vi "XNETDB.Add.vi"(8 "error in (no error)":errorcluster, 11 "Databases Section Ref":T1 format="%.0x") -> (0 "error out":errorcluster, 3 "Databases Section Ref":u64)   [LabVIEW 2019, in "Diagnostics Addon Shared.lvlib"]
uses:
  Diagnostics Addon Shared.lvlib
  <vilib>/NI VeriStand/Custom Device API/Custom Device Item Ref.ctl
  Constants.vi
  <vilib>/NI/NI VeriStand Advanced SysDef API/_SubVIs/SysDef.Property.Set.String.vi
  <vilib>/NI/NI VeriStand Advanced SysDef API/SysDef API/Advanced System Definition.lvlib
  <vilib>/NI VeriStand/Custom Device API/Custom Device API.lvlib
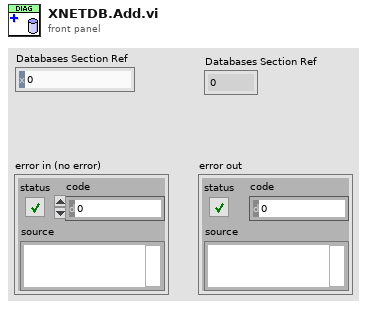
[diagram p1: front panel]
types:
  T1 = typedef "Custom Device API.lvlib/Custom Device Item Ref.ctl" = u64
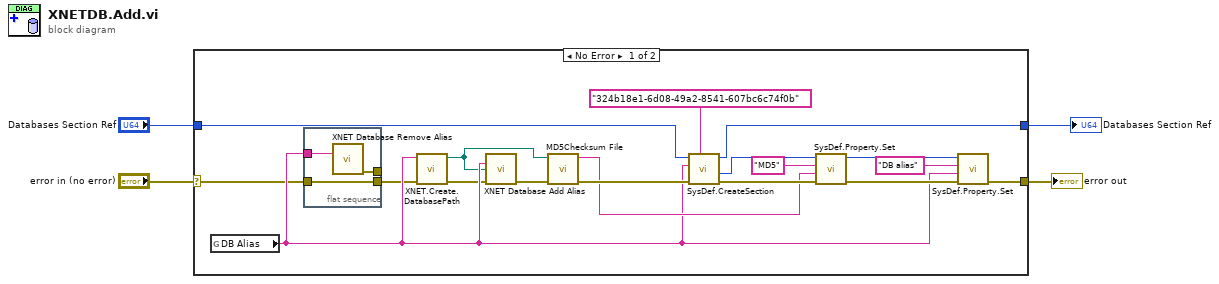
[diagram p0: block diagram]
diagram:
  n1 = case shown="No Error" "error in (no error)" {
    selector: "error in (no error)" -> [w6 w27]
    tunnel: "Databases Section Ref" -> [w22 w26]
    tunnel: [w21 w27] -> w3
    tunnel: [w5 w26] -> w1
    frame No Error {
      n2 = global read "Constants.vi" "DB Alias"() -> (w10:string)
      n3 = flat-sequence {
        tunnel: [w25] -> w8
        tunnel: w6 -> [w25]
        tunnel: [w24] -> _
        tunnel: w10 -> [w23]
        frame #0 {
          n4 = call <vilib>:"XNET Database Remove Alias.vi"("alias"=w23) -> ("error out"=w24:errorcluster)  [unwired: 14 in]
        }
      }
      n5 = call "XNET.Create.DatabasePath.vi"("error in (no error)"=w8, "DB Alias"=w10) -> ("error out"=w9:errorcluster, "DB Path"=w7:path)  [unwired: 8 in]
      n6 = call <vilib>:"XNET Database Add Alias.vi"("alias"=w10, "filepath"=w7, "error in (no error)"=w9) -> ("error out"=w20:errorcluster)  [unwired: 12 in]
      n7 = call <vilib>:"MD5Checksum File.vi"("error in (no error)"=w20, "Path"=w7) -> ("error out"=w12:errorcluster, "MD5 message-digest"=w11:string)  [unwired: 8 in]
      n8 = call <vilib>:"SysDef.CreateSection.vi"("GUID"="324b18e1-6d08-49a2-8541-607bc6c74f0b" ("GUID (Default Section)"), "error in (no error)"=w12, "Name"=w10, "nodeID"=w22) -> ("error out"=w18:errorcluster, "New NodeID"=w19:u64, "nodeID out"=w5:u64)  [unwired: 4 in, 1 out]
      n9 = call-poly <vilib>:"SysDef.Property.Set.vi"("error in (no error)"=w18, "Value"=w11, "Property Name"="MD5", "nodeID"=w19) -> ("error out"=w17:errorcluster, "nodeID out"=w16:u64)  [unwired: 6 in]
      n10 = call-poly <vilib>:"SysDef.Property.Set.vi"("error in (no error)"=w17, "Value"=w10, "Property Name"="DB alias", "nodeID"=w16) -> ("error out"=w21:errorcluster)  [unwired: 6 in, 1 out]
    }
    frame Error {
    }
  }
  "error out" <- w3
  "Databases Section Ref" <- w1
